vi "PR_screw_eve_result.vi"(6 "結果":string, 8 "數據":string, 9 "data":T1, 10 "barcode":string="984132195", 11 "DBlink":string="Driver={ODBC Driver 17 for SQL Server};Server=localhost\\SQLEXPRESS;Database=ZDX201;UID=labview;PWD=Dsa@54137926") -> ()   [LabVIEW 2019]
panel:
  out "error out":errorcluster
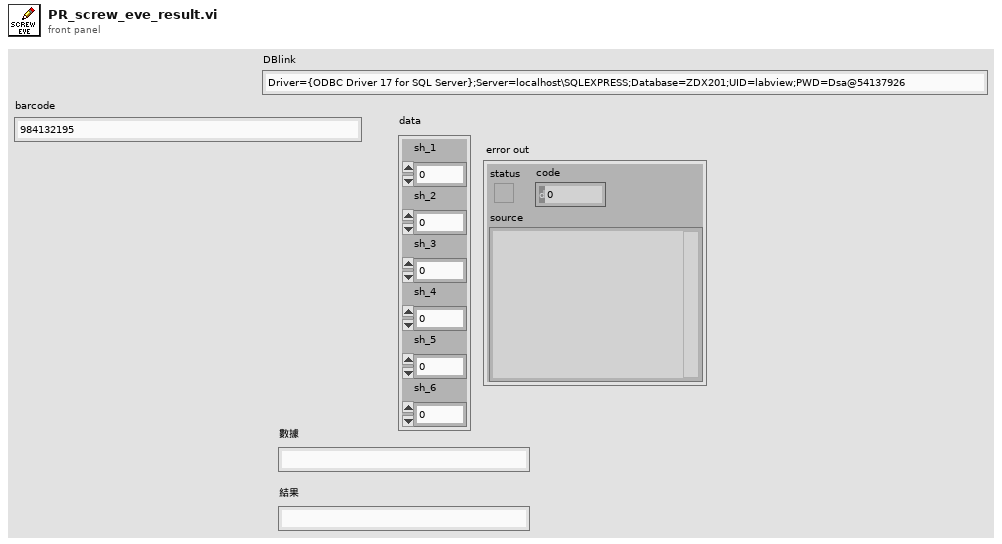
[diagram p1: front panel]
types:
  T1 = cluster{"sh_1":dbl, "sh_2":dbl, "sh_3":dbl, "sh_4":dbl, "sh_5":dbl, "sh_6":dbl}
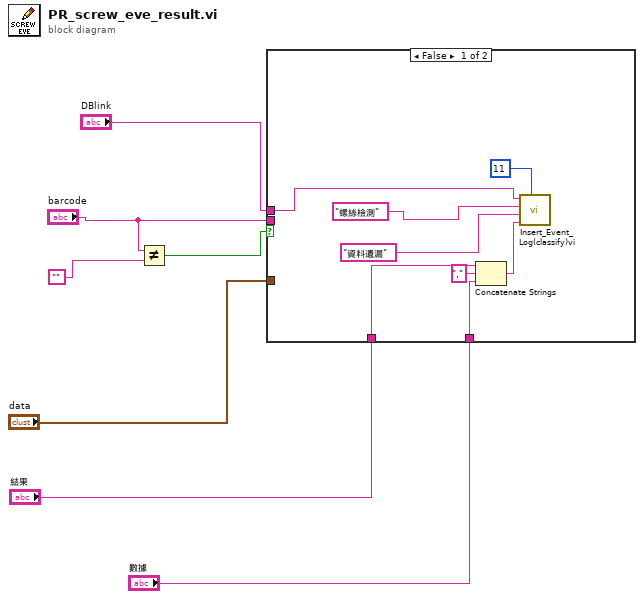
[diagram p0: block diagram]
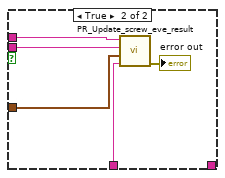
[diagram p2: hidden frame]
diagram:
  n1 = Not Equal?(x="barcode", y="") -> (x != y?=w4:bool)
  n2 = case shown="False" w4 {
    tunnel: "DBlink" -> [w12 w20]
    tunnel: "barcode" -> [_ w19]
    tunnel: "結果" -> [w11 w18]
    tunnel: "data" -> [_ w17]
    tunnel: "數據" -> [w8 _]
    frame False {
      n3 = Concatenate Strings(w11, "," ("string"), w8) -> (w9:string)
      n4 = call "Insert_Event_Log(classify)vi.vi"("classify"=i16 11, "data"=w9, "message"="資料遺漏", "id"="螺絲檢測", "DBlink"=w12) -> ()  [unwired: 6 in, 1 out]
    }
    frame True {
      n5 = call "PR_Update_screw_eve_result.vi"("result"=w18, "data"=w17, "barcode"=w19, "DBlink"=w20) -> ("error out"=→"error out":errorcluster)  [unwired: 7 in]
    }
  }
